vi "MoveXY.vi"(8 "error in (no error)":errorcluster, 10 "XY Cluster":T1 {"Y Position (0 units)" format="%.6f"; "X Position (0 units)" format="%.6f"}, 11 "VISA resource name":refnum<visa-resource-name>) -> (0 "error out":errorcluster, 3 "VISA resource Out":refnum<visa-resource-name>)   [LabVIEW 2015]
uses:
  <userlib>/Newport ESP301/Newport ESP301.lvlib
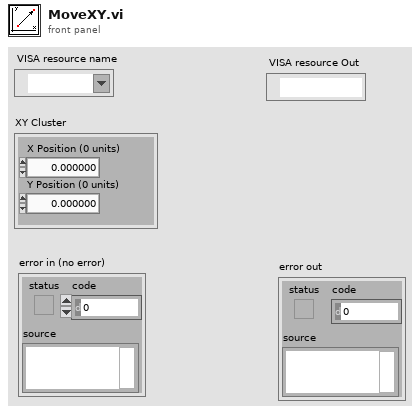
[diagram p1: front panel]
types:
  T1 = cluster{"X Position (0 units)":dbl, "Y Position (0 units)":dbl}
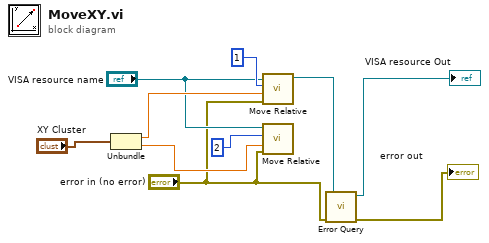
[diagram p0: block diagram]
diagram:
  n1 = Unbundle("XY Cluster") -> ("X Position (0 units)"=w7:dbl, "Y Position (0 units)"=w6:dbl)
  n2 = call <userlib>:"Move Relative.vi"("error in (no error)"="error in (no error)", "Position (0 units)"=w7, "Axis (1)"=1, "VISA resource name"="VISA resource name") -> ("VISA resource name out"=w3:refnum<visa-resource-name>)  [unwired: 2 in, 1 out]
  n3 = call <userlib>:"Move Relative.vi"("error in (no error)"="error in (no error)", "Position (0 units)"=w6, "Axis (1)"=2, "VISA resource name"="VISA resource name") -> ()  [unwired: 2 in, 2 out]
  n4 = call <userlib>:"Error Query.vi"("error in (no error)"="error in (no error)", "VISA resource name"=w3) -> ("error out"=→"error out":errorcluster, "VISA resource name out"=→"VISA resource Out":refnum<visa-resource-name>)  [unwired: 2 in, 2 out]
